vi "SharedVariables_init.vi"(8 "error in (no error)":errorcluster) -> (0 "error out":errorcluster)   [LabVIEW 2013]
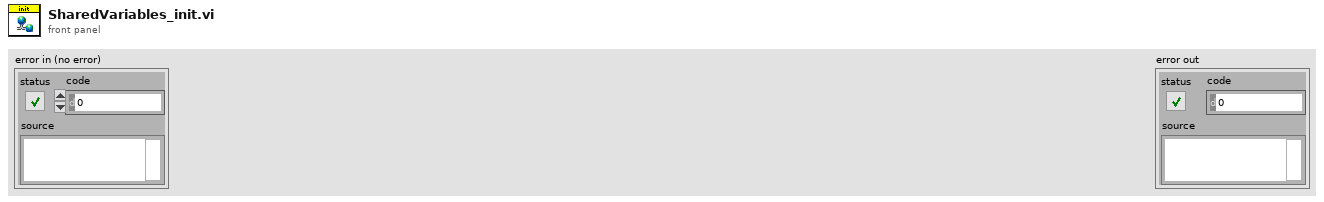
[diagram p1: front panel]
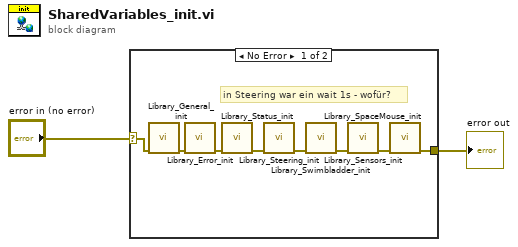
[diagram p0: block diagram]
diagram:
  n1 = case shown="No Error" "error in (no error)" {
    selector: "error in (no error)" -> [w5 w11]
    tunnel: [w6 w11] -> w2
    frame No Error {
      # "in Steering war ein wait 1s - wofür?"
      n2 = call "Library_General_init.vi"("error in (no error)"=w5) -> ("error out"=w4:errorcluster)  [unwired: 10 in]
      n3 = call "Library_Error_init.vi"("error in (no error)"=w4) -> ("error out"=w3:errorcluster)  [unwired: 10 in]
      n4 = call "Library_Status_init.vi"("error in (no error)"=w3) -> ("error out"=w10:errorcluster)  [unwired: 10 in]
      n5 = call "Library_Steering_init.vi"("error in (no error)"=w10) -> ("error out"=w9:errorcluster)  [unwired: 10 in]
      n6 = call "Library_Swimbladder_init.vi"("error in (no error)"=w9) -> ("error out"=w8:errorcluster)  [unwired: 10 in]
      n7 = call "Library_Sensors_init.vi"("error in (no error)"=w8) -> ("error out"=w7:errorcluster)  [unwired: 10 in]
      n8 = call "Library_SpaceMouse_init.vi"("error in (no error)"=w7) -> ("error out"=w6:errorcluster)  [unwired: 10 in]
    }
    frame Error {
    }
  }
  "error out" <- w2
